vi "setMeasurementTimingBudget.vi"(8 "error in":errorcluster, 9 "budget_us":u32, 10 "Slave Address (7-bit)":u8, 11 "I2C Ref In":T1) -> (0 "error out":errorcluster, 2 "status":bool, 3 "I2C Ref Out":T1)   [LabVIEW 2018]
uses:
  <vilib>/myRIO/Instrument Drivers/Onboard IO/I2C/typedefs/I2C Reference.ctl
  <vilib>/myRIO/Common/Instrument Driver Framework/Utilities/typedefs/myRIO Generic Hardware Reference.ctl
  <vilib>/myRIO/Common/Instrument Driver Framework/Utilities/typedefs/Hardware Version Enum.ctl
  <vilib>/myRIO/Common/Instrument Driver Framework/Utilities/typedefs/myRIO v1.0 Reference.ctl
  <vilib>/myRIO/Common/Instrument Driver Framework/Utilities/typedefs/Generic FPGA Reference.ctl
  <vilib>/myRIO/Common/Instrument Driver Framework/myRIO v1.0/I2C/typedefs/I2C Channels Enum.ctl
  <vilib>/myRIO/Instrument Drivers/Onboard IO/I2C/typedefs/I2C Configuration.ctl
  <vilib>/myRIO/Instrument Drivers/Onboard IO/I2C/typedefs/I2C Transfer Rate.ctl
  <vilib>/Utility/error.llb/Error Cluster From Error Code.vi
  <vilib>/myRIO/Common/Instrument Driver Framework/myRIO v1.0/I2C/vis/myRIO v1.0 Write I2C.vi
  <vilib>/myRIO/Instrument Drivers/Onboard IO/I2C/I2C.lvlib
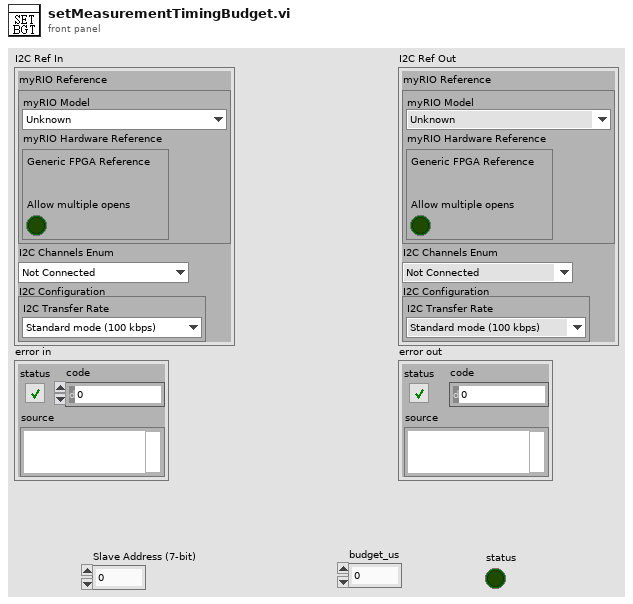
[diagram p1: front panel]
types:
  T1 = typedef "I2C.lvlib/I2C Reference.ctl" = cluster{"myRIO Reference":T2, "I2C Channels Enum":T6, "I2C Configuration":T7}
  T2 = typedef "myRIO Generic Hardware Reference.ctl" = cluster{"myRIO Model":T3, "myRIO Hardware Reference":T4}
  T3 = typedef "Hardware Version Enum.ctl" = enum16{"Unknown", "myRIO-1900", "myRIO-1950", "roboRIO", "NI ELVIS RIO CM", "ELVIS III"}
  T4 = typedef "myRIO v1.0 Reference.ctl" = cluster{"Generic FPGA Reference":T5, "Allow multiple opens":bool}
  T5 = typedef "Generic FPGA Reference.ctl" = refnum<k20>
  T6 = typedef "I2C Channels Enum.ctl" = enum16{"Not Connected", "A/I2C", "B/I2C", "I2C/I2C"}
  T7 = typedef "I2C.lvlib/I2C Configuration.ctl" = cluster{"I2C Transfer Rate":T8}
  T8 = typedef "I2C.lvlib/I2C Transfer Rate.ctl" = enum16{"Standard mode (100 kbps)", "Fast mode (400 kbps)"}
  T9 = cluster{"tcc":bool, "dss":bool, "msrc":bool, "pre_range":bool, "final_range":bool}
  T10 = cluster{"pre_range_vcsel_period_pclks":u16, "final_range_vcsel_period_pclks":u16, "msrc_dss_tcc_mclks":u16, "pre_range_mclks":u16, "final_range_mclks":u16, "msrc_dss_tcc_us":u32, "pre_range_us":u32, "final_range_us":u32}
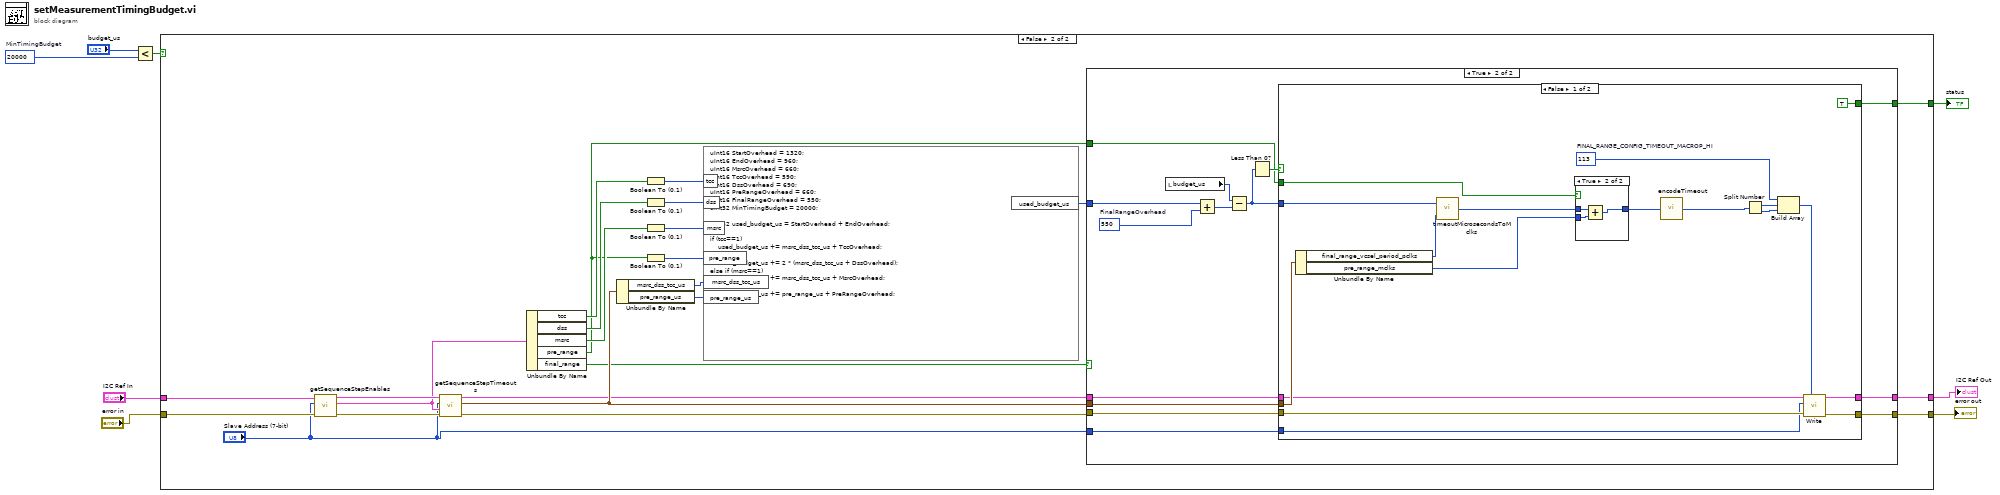
[diagram p0: block diagram]
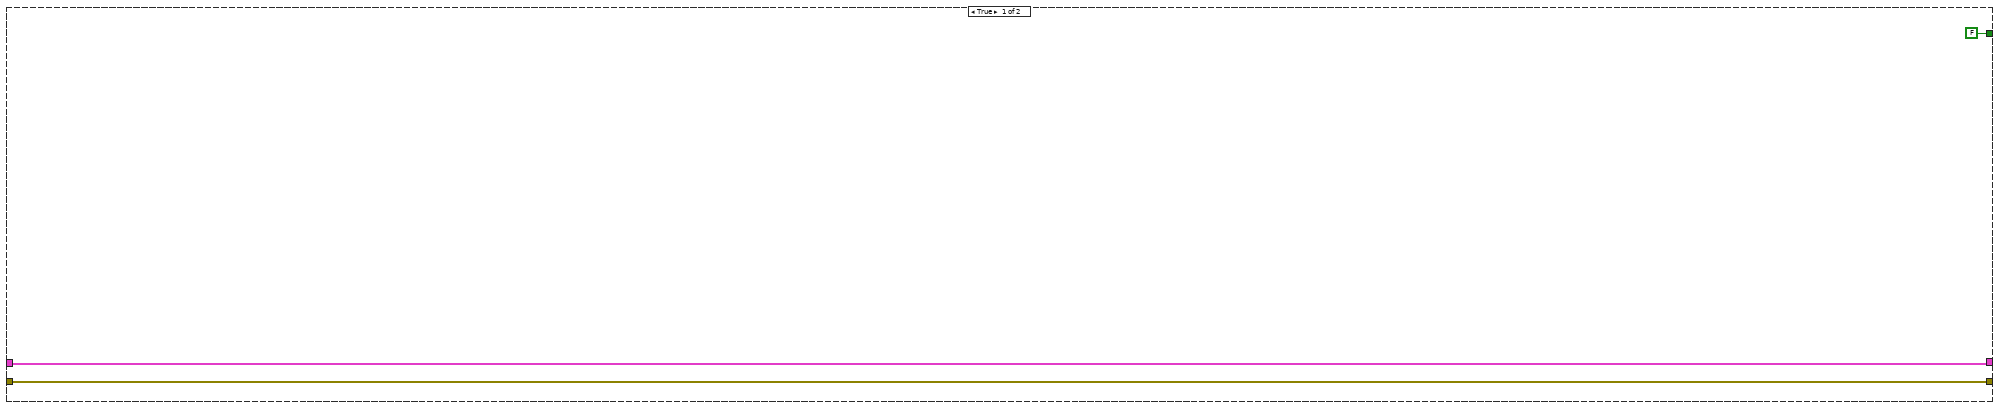
[diagram p2: hidden frame]
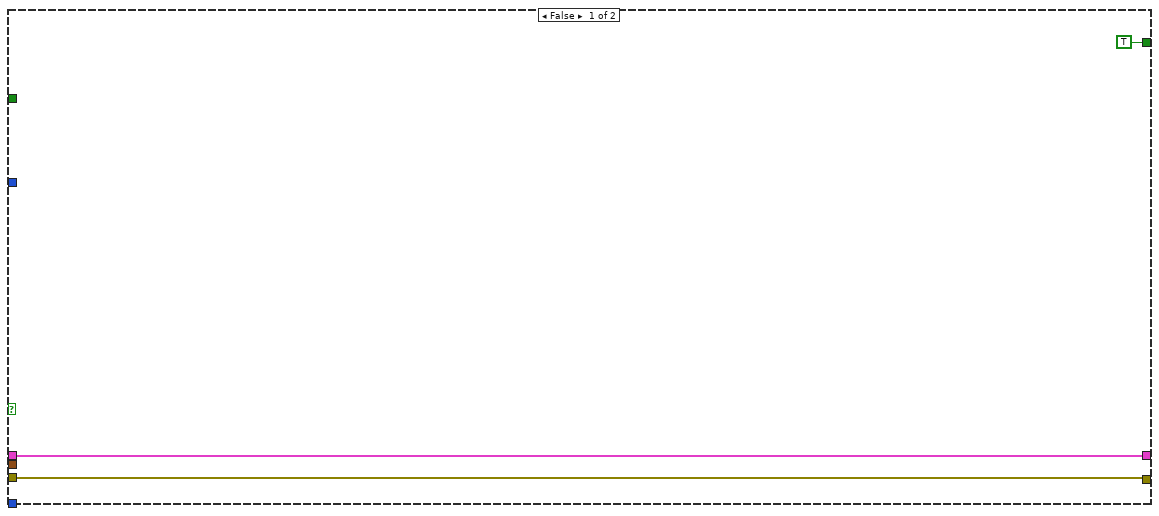
[diagram p3: hidden frame]
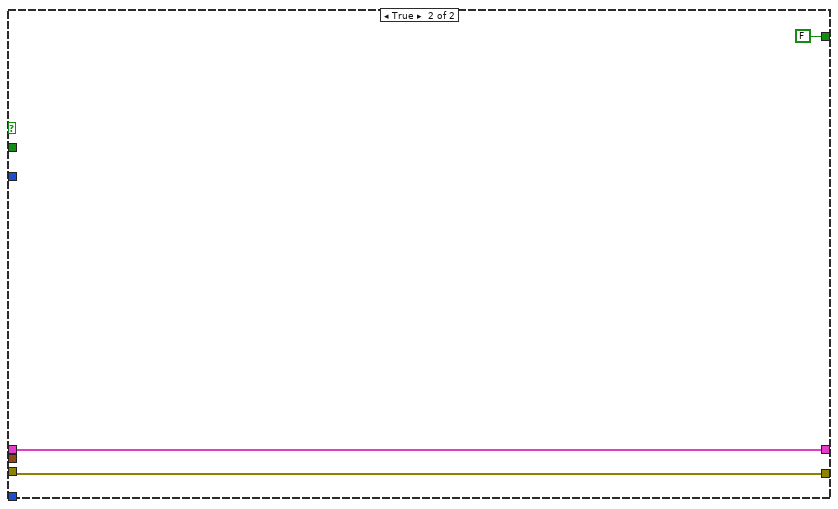
[diagram p5: hidden frame]
diagram:
  w7 = u32 20000  # MinTimingBudget
  n1 = Less?(x="budget_us", y=w7) -> (x < y?=w6:bool)
  n2 = case shown="False" w6 {
    tunnel: [FALSE w24] -> w5
    tunnel: "I2C Ref In" -> [w10 w18]
    tunnel: "error in" -> [w9 w17]
    tunnel: [w9 w13] -> w2
    tunnel: [w10 w12] -> w1
    frame True {
    }
    frame False {
      n3 = call "getSequenceStepEnables.vi"("error in"=w17, "Slave Address (7-bit)"="Slave Address (7-bit)", "I2C Ref In"=w18) -> ("error out"=w35:errorcluster, "enables"=w22:T9, "I2C Ref Out"=w34:T1)  [unwired: 6 in]
      n4 = call "getSequenceStepTimeouts.vi"("error in"=w35, "enables"=w22, "Slave Address (7-bit)"="Slave Address (7-bit)", "I2C Ref In"=w34) -> ("error out"=w15:errorcluster, "timeouts"=w21:T10, "I2C Ref Out"=w16:T1)  [unwired: 4 in]
      n5 = Unbundle By Name(w22) -> ("tcc"=w33:bool, "dss"=w32:bool, "msrc"=w31:bool, "pre_range"=w19:bool, "final_range"=w20:bool)
      n6 = Unbundle By Name(w21) -> ("msrc_dss_tcc_us"=w26:u32, "pre_range_us"=w25:u32)
      n7 = Boolean To (0,1)(Boolean=w33) -> (0, 1=w30:i16)
      n8 = Boolean To (0,1)(Boolean=w32) -> (0, 1=w29:i16)
      n9 = Boolean To (0,1)(Boolean=w31) -> (0, 1=w28:i16)
      n10 = Boolean To (0,1)(Boolean=w19) -> (0, 1=w27:i16)
      n11 = formula code="uInt16 StartOverhead = 1320; \nuInt16 EndOverhead = 960;\nuInt16 MsrcOverhead = 660;\nuInt16 TccOverhead = 590;\nuInt16 DssOverhead = 690;\nuInt16 PreRangeOverhead = 660;\nuInt16 FinalRangeOverhead = 550;\nuInt32 MinTimingBudget = 20000;\n\nuInt32 used_budget_us = StartOverhead + EndOverhead;\n\nif (tcc==1)\n    used_budget_us += msrc_dss_tcc_us + TccOverhead;\nif (dss==1)\n    used_budget_us += 2 * (msrc_dss_tcc_us + DssOverhead);\nelse if (msrc==1)\n    used_budget_us += msrc_dss_tcc_us + MsrcOverhead;\nif (pre_range==1)\n    used_budget_us += pre_range_us + PreRangeOverhead;"("tcc"=w30, "dss"=w29, "msrc"=w28, "pre_range"=w27, "pre_range_us"=w25, "msrc_dss_tcc_us"=w26) -> ("used_budget_us"=w23:u32)
      n12 = case shown="True" w20 {
        tunnel: [TRUE w50] -> w24
        tunnel: w23 -> [_ w52]
        tunnel: w19 -> [_ w45]
        tunnel: w21 -> [_ w44]
        tunnel: w16 -> [w37 w43]
        tunnel: w15 -> [w36 w42]
        tunnel: "Slave Address (7-bit)" -> [_ w41]
        tunnel: [w36 w40] -> w13
        tunnel: [w37 w39] -> w12
        frame False {
        }
        frame True {
          w51 = u16 550  # FinalRangeOverhead
          n13 = local read "budget_us"() -> (w49:u32)
          n14 = Add(x=w52, y=w51) -> (x+y=w48:u32)
          n15 = Subtract(x=w49, y=w48) -> (x-y=w46:u32)
          n16 = Less Than 0?(x=w46) -> (x < 0?=w47:bool)
          n17 = case shown="False" w47 {
            tunnel: [TRUE FALSE] -> w50
            tunnel: w46 -> [w70 _]
            tunnel: w45 -> [w69 _]
            tunnel: w44 -> [w68 _]
            tunnel: w43 -> [w58 w76]
            tunnel: w42 -> [w57 w75]
            tunnel: w41 -> [w56 _]
            tunnel: [w55 w75] -> w40
            tunnel: [w54 w76] -> w39
            frame False {
              w64 = u8 113  # FINAL_RANGE_CONFIG_TIMEOUT_MACROP_HI
              n18 = Unbundle By Name(w68) -> ("final_range_vcsel_period_pclks"=w67:u16, "pre_range_mclks"=w66:u16)
              n19 = call "timeoutMicrosecondsToMclks.vi"("vcsel_period_pclks"=w67, "timeout_period_us"=w70) -> ("timeout_period_mclks"=w65:u32)
              n20 = case shown="True" w69 {
                tunnel: w66 -> [_ w74]
                tunnel: w65 -> [w71 w73]
                tunnel: [w71 w72] -> w53
                frame False {
                }
                frame True {
                  n21 = Add(x=w73, y=w74) -> (x+y=w72:u32)
                }
              }
              n22 = call "encodeTimeout.vi"("timeout_mclks"=w53) -> ("reg_val"=w62:u16)
              n23 = Split Number(x=w62) -> (hi(x)=w61:u8, lo(x)=w60:u8)
              n24 = Build Array(w64, w61, w60) -> (w63:u8[])
              n25 = call <vilib>:"Write.vi"("error in (no error)"=w57, "Bytes to Write"=w63, "Slave Address (7-bit)"=w56, "I2C Ref In"=w58) -> ("error out"=w55:errorcluster, "I2C Ref Out"=w54:T1)  [unwired: 6 in]
            }
            frame True {
            }
          }
        }
      }
    }
  }
  "status" <- w5
  "I2C Ref Out" <- w1
  "error out" <- w2
